vi "Set Acquisition Mode.vi"(8 "error in (no error)":errorcluster, 11 "mode":i32) -> (0 "error out":errorcluster, 3 "function return":u32)   [LabVIEW 2018, in "AndorSDK.lvlib"]
doc: "EXPNETTYPE unsigned int WINAPI SetAcquisitionMode(int mode);"
uses:
  AndorSDK.lvlib
  ATMCD32D.dll
  OwnVIs/AndorOWN.lvlib
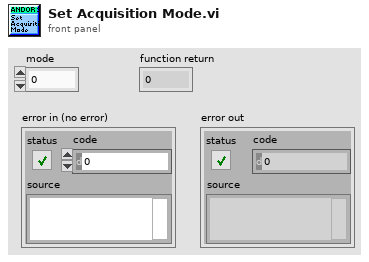
[diagram p1: front panel]
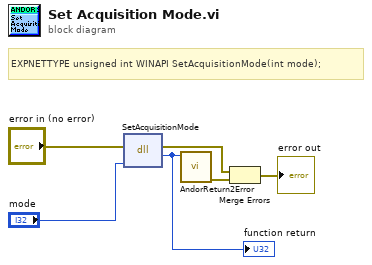
[diagram p0: block diagram]
diagram:
  # "EXPNETTYPE unsigned int WINAPI SetAcquisitionMode(int mode);"
  n1 = dll-call lib="C:/Users/e14user/Documents/LabVIEW software/GitRepo/lib/ANDOR/Andor SDK/ATMCD32D.*" fn="SetAcquisitionMode"(error in="error in (no error)", "mode"="mode") -> (error out=w3:errorcluster, w1:u32)  [unwired: 3 in, 1 out]
  "function return" <- w1
  n2 = call "AndorReturn2Error.vi"("Camera return"=w1) -> ("error out"=w2:errorcluster)  [unwired: 10 in]
  n3 = Merge Errors(w3, w2) -> (→"error out":errorcluster)
